vi "Popout Subpanel.vi"(8 "error in (no error)":errorcluster, 10 "Sub Panel":refnum<vi>, 11 "PanelManager in":refnum<class "PanelManager.lvclass">) -> (0 "error out":errorcluster, 3 "PanelManager out":refnum<class "PanelManager.lvclass">)   [LabVIEW 2018, in "OOPanel.lvlib" / "PanelManager.lvclass"]
uses:
  PanelManager.lvclass
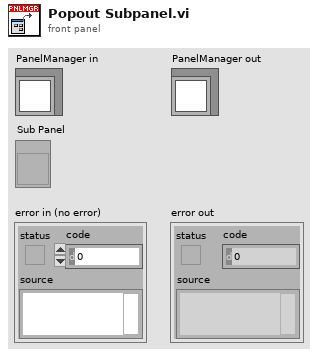
[diagram p1: front panel]
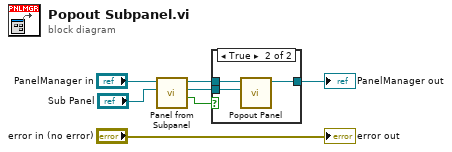
[diagram p0: block diagram]
diagram:
  n1 = call "Panel from Subpanel.vi"("Sub Panel"="Sub Panel", "PanelManager in"="PanelManager in") -> ("Has Panel?"=w1:bool, "Panel"=w3:refnum<class "Panel.lvclass">, "PanelManager out"=w2:refnum<class "PanelManager.lvclass">)  [unwired: 6 in, 1 out]
  n2 = case shown="True" w1 {
    tunnel: [w8 w11] -> w6
    tunnel: w3 -> [_ w10]
    tunnel: w2 -> [w8 w9]
    frame False {
    }
    frame True {
      n3 = call "Popout Panel.vi"("Panel"=w10, "PanelManager in"=w9) -> ("PanelManager out"=w11:refnum<class "PanelManager.lvclass">)  [unwired: 8 in, 1 out]
    }
  }
  "PanelManager out" <- w6
  "error out" <- "error in (no error)"
